vi "WaitState.vi"(7 "Enum输入":refnum<vi>, 8 "错误输入（无错误）":errorcluster, 10 "™z²é î‘B":T1=enum."Idle") -> (0 "错误输出":errorcluster)   [LabVIEW 2012]
uses:
  SystemState.ctl
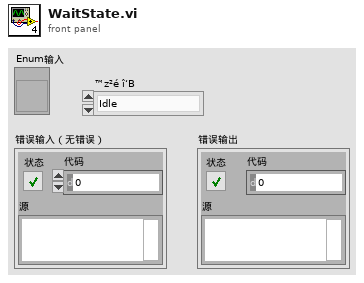
[diagram p1: front panel]
types:
  T1 = typedef "SystemState.ctl" = enum16{"Pause", "Quit", "Error", "Stopping", "Starting", "Init", "Scan", "Menu", "ReadConf", "Idle"}
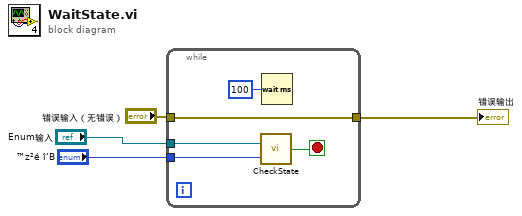
[diagram p0: block diagram]
diagram:
  n1 = while {
    tunnel: "Enum输入" -> [w9]
    tunnel: "错误输入（无错误）" -> [w7]
    tunnel: [w7] -> w3
    tunnel: "™z²é î‘B" -> [w5]
    stop <- w8 stop-if-true
    n2 = call "CheckState.vi"("™z²é î‘B"=w5, "Ïµ½y î‘B"=w9) -> ("ChkOK?"=w8:bool)
    n3 = Wait (ms)(milliseconds to wait=u32 100 ("等待时间（毫秒）")) -> ()  [unwired: 1 out]
  }
  "错误输出" <- w3
